vi "Sigma_Serial read with time out.vi"(0 "VISA resource name":refnum<visa-resource-name>, 7 "Time out":dbl=1.0, 9 "Byte to read":u32=2, 11 "error in (no error)":errorcluster) -> (4 "VISA resource name out":refnum<visa-resource-name>, 6 "read buffer":string, 8 "Time out":bool, 15 "error out":errorcluster)   [LabVIEW 2018]
panel:
  out "Serial Settings:Number of Bytes at Serial Port":u32
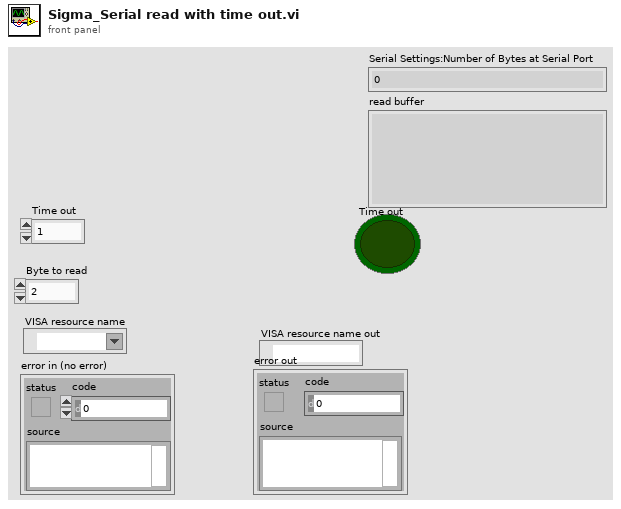
[diagram p1: front panel]
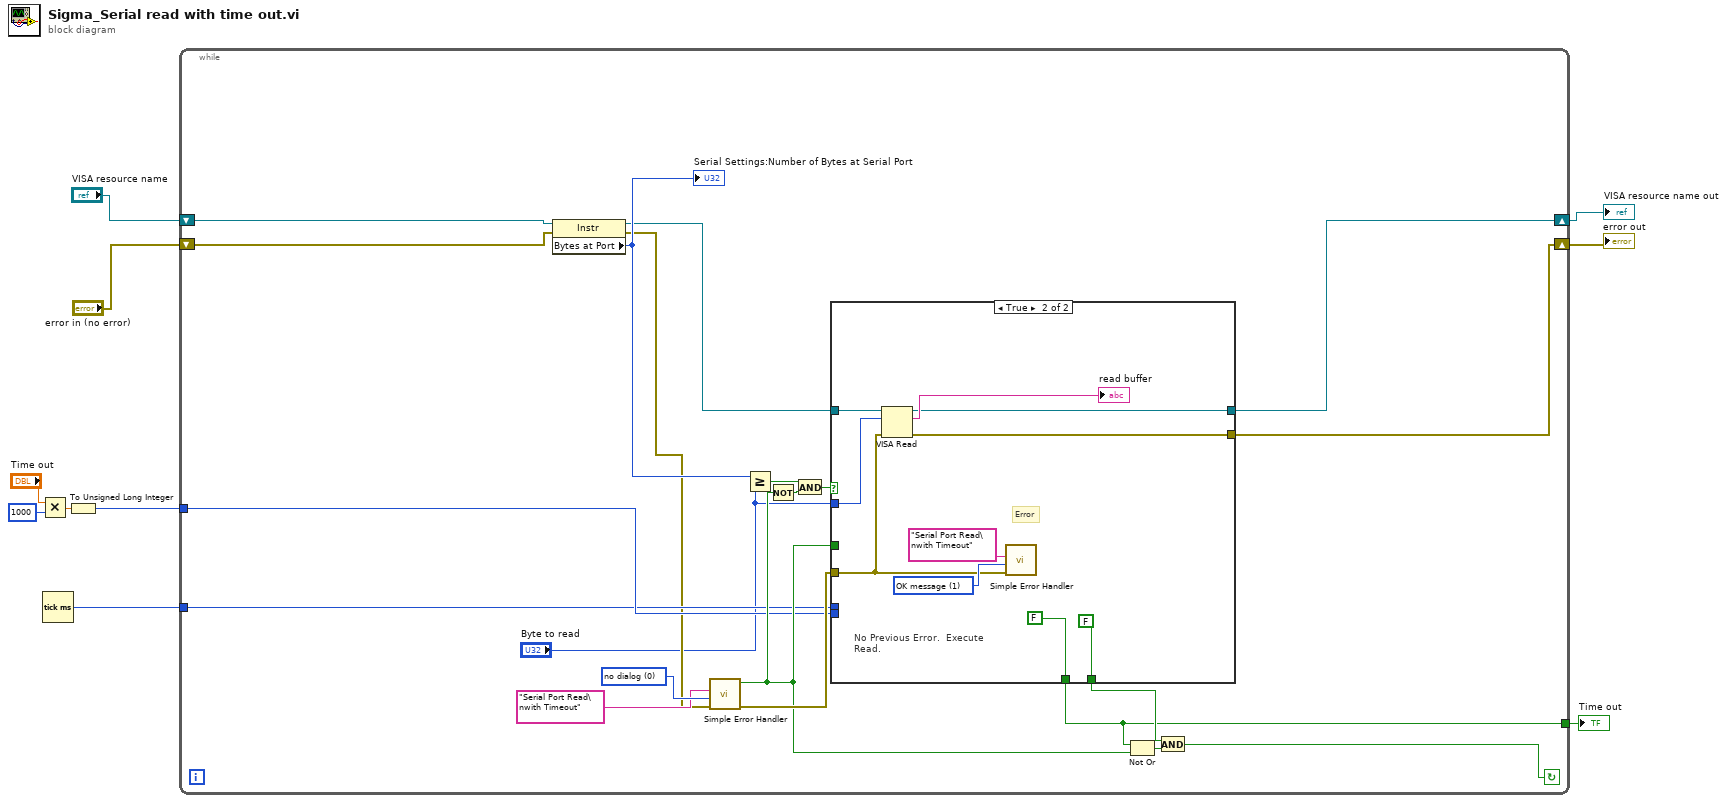
[diagram p0: block diagram]
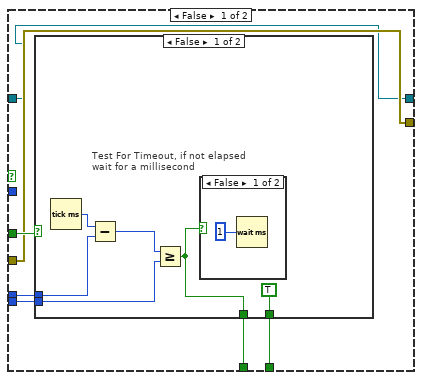
[diagram p2: hidden frame]
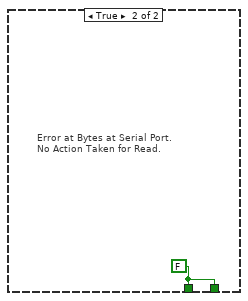
[diagram p4: hidden frame]
diagram:
  n1 = Multiply(x="Time out", y=u32 1000) -> (x*y=w9:dbl)
  n2 = Tick Count (ms)() -> (millisecond timer value=w7:u32)
  n3 = To Unsigned Long Integer(number=w9) -> (unsigned 32bit integer=w8:u32)
  n4 = while {
    tunnel: w8 -> [w22]
    tunnel: w7 -> [w21]
    tunnel: [w17] -> w1
    shift-right: [w13] -> w4
    shift-left: "error in (no error)" -> [w15]
    shift-right: [w12] -> w3
    shift-left: "VISA resource name" -> [w16]
    stop <- w18 continue-if-true
    w27 = 0 items=["no dialog", "OK message", "continue or stop message"] ("type of dialog (OK msg:1)")
    n5 = property class="Instr"(reference=w16, error in=w15) -> (reference out=w14:refnum<visa-resource-name>, error out=w19:errorcluster, "Bytes at Port"=w20:u32)
    "Serial Settings:Number of Bytes at Serial Port" <- w20
    n6 = call <vilib>:"Simple Error Handler.vi"("error source (\" \")"="Serial Port Read\nwith Timeout", "type of dialog (OK msg:1)"=w27, "error in (no error)"=w19) -> ("error?"=w23:bool, "error out"=w28:errorcluster)  [unwired: 1 in, 4 out]
    n7 = Greater Or Equal?(x=w20, y="Byte to read") -> (x >= y?=w30:bool)
    n8 = Not(x=w23) -> (.not. x?=w29:bool)
    n9 = And(x=w30, y=w29) -> (x .and. y?=w31:bool)
    n10 = case shown="True" w31 {
      tunnel: "Byte to read" -> [_ w48]
      tunnel: w23 -> [w36 _]
      tunnel: w28 -> [w33 w50]
      tunnel: [w38 FALSE] -> w24
      tunnel: w21 -> [w37 _]
      tunnel: [w35 FALSE] -> w17
      tunnel: w22 -> [w34 _]
      tunnel: w14 -> [w32 w51]
      tunnel: [w33 w49] -> w13
      tunnel: [w32 w47] -> w12
      frame False {
        n11 = case shown="False" w36 {
          tunnel: [TRUE w46] -> w38
          tunnel: w37 -> [w42 _]
          tunnel: [w41 w46] -> w35
          tunnel: w34 -> [w39 _]
          frame False {
            # "Test For Timeout, if not elapsed\nwait for a millisecond"
            n12 = Tick Count (ms)() -> (millisecond timer value=w43:u32)
            n13 = Subtract(x=w43, y=w42) -> (x-y=w40:u32)
            n14 = Greater Or Equal?(x=w40, y=w39) -> (x >= y?=w41:bool)
            n15 = case shown="False" w41 {
              frame False {
                n16 = Wait (ms)(milliseconds to wait=u32 1 ("f")) -> ()  [unwired: 1 out]
              }
              frame True {
              }
            }
          }
          frame True {
            w46 = FALSE
            # "Error at Bytes at Serial Port.\nNo Action Taken for Read."
          }
        }
      }
      frame True {
        w53 = 1 items=["no dialog", "OK message", "continue or stop message"] ("type of dialog (OK msg:1)")
        # "No Previous Error.  Execute\nRead."
        # "Error"
        n17 = VISA Read(VISA resource name=w51, byte count=w48, error in (no error)=w50) -> (VISA resource name out=w47:refnum<visa-resource-name>, read buffer=→"read buffer":string, error out=w49:errorcluster)  [unwired: 1 out]
        n18 = call <vilib>:"Simple Error Handler.vi"("error source (\" \")"="Serial Port Read\nwith Timeout", "type of dialog (OK msg:1)"=w53, "error in (no error)"=w50) -> ()  [unwired: 1 in, 6 out]
      }
    }
    n19 = Not Or(1:w23, 2:w17) -> (0:w25:bool)
    n20 = And(x=w24, y=w25) -> (x .and. y?=w18:bool)
  }
  "VISA resource name out" <- w3
  "error out" <- w4
  "Time out" <- w1
